vi "XYGraph.vi"() -> ()   [LabVIEW 2015]
panel:
  in  "Dato A":dbl
  out "XY Graph 2":cluster{dbl[], dbl[]}(graph)
  out "XY Graph":cluster{i32[], dbl[]}[](graph)
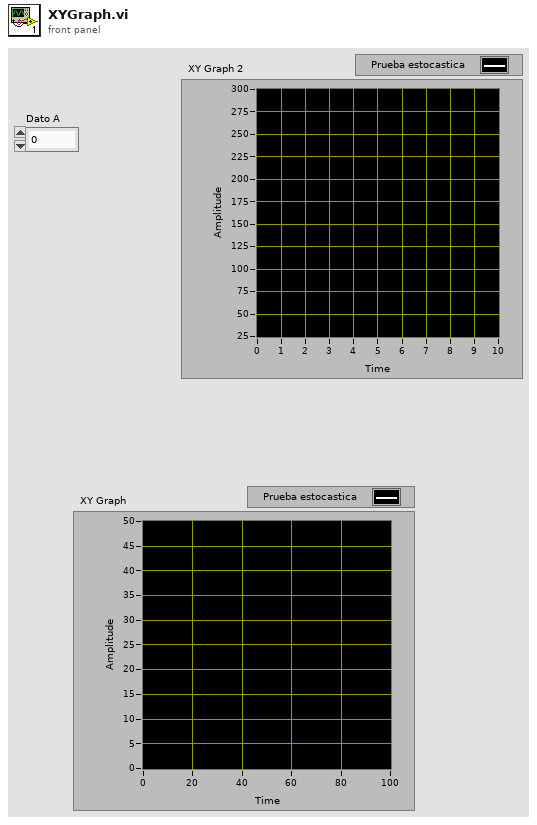
[diagram p1: front panel]
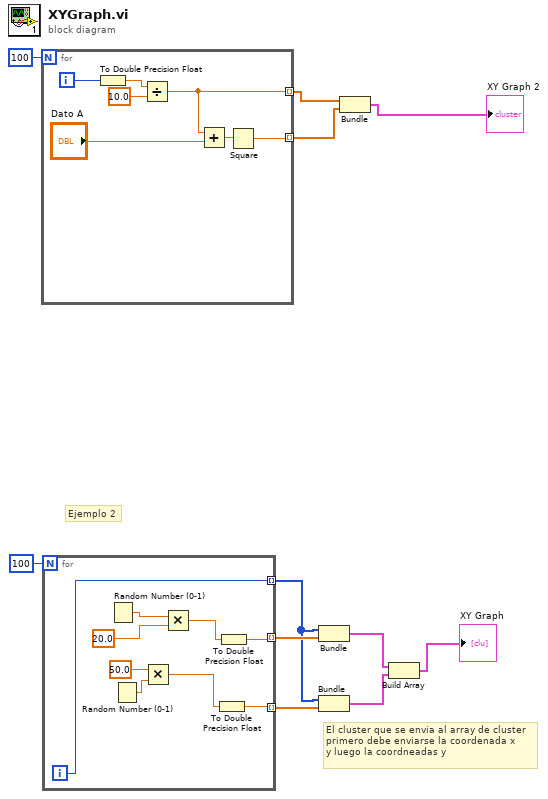
[diagram p0: block diagram]
diagram:
  # "Ejemplo 2"
  # "El cluster que se envia al array de cluster\nprimero debe enviarse la coordenada x \ny luego la coordneadas y"
  n1 = for {
    N: 100 -> [_]
    tunnel: [w14] -> w3 mode=indexing
    tunnel: [w12] -> w2 mode=indexing
    i -> [w18]
    n2 = To Double Precision Float(number=w18) -> (double precision float=w16:dbl)
    n3 = Divide(x=w16, y=10.0) -> (x/y=w14:dbl)
    n4 = Add(x=w14, y="Dato A") -> (x+y=w13:dbl)
    n5 = Square(x=w13) -> (x^2=w12:dbl)
  }
  n6 = for {
    N: 100 -> [_]
    tunnel: [w24] -> w9 mode=indexing
    tunnel: [w20] -> w10 mode=indexing
    tunnel: [w23] -> w8 mode=indexing
    i -> [w24]
    n7 = Random Number (0-1)() -> (number: 0 to 1=w27:dbl)
    n8 = Random Number (0-1)() -> (number: 0 to 1=w25:dbl)
    n9 = Multiply(x=50.0, y=w25) -> (x*y=w22:dbl)
    n10 = Multiply(x=w27, y=20.0) -> (x*y=w21:dbl)
    n11 = To Double Precision Float(number=w22) -> (double precision float=w23:dbl)
    n12 = To Double Precision Float(number=w21) -> (double precision float=w20:dbl)
  }
  n13 = Bundle(w9, w10) -> (w6:cluster{i32[], dbl[]})  [unwired: 1 in]
  n14 = Bundle(w9, w8) -> (w7:cluster{i32[], dbl[]})  [unwired: 1 in]
  n15 = Bundle(w3, w2) -> (→"XY Graph 2":cluster{dbl[], dbl[]})  [unwired: 1 in]
  n16 = Build Array(w6, w7) -> (→"XY Graph":cluster{i32[], dbl[]}[])
